vi "GetData.vi"(8 "error in (no error)":errorcluster caption="Fehler (Eingang, kein Fehler)", 10 "Name":string, 11 "Dictionary Eingang":refnum<class "Dictionary.lvclass"> caption="DNL_LabVIEW Object in") -> (0 "error out":errorcluster caption="Fehler (Ausgang)", 2 "Wert":variant, 3 "Dictionary Ausgang":refnum<class "Dictionary.lvclass"> caption="DNL_LabVIEW Object out")   [LabVIEW 2013, in "Dictionary.lvclass"]
uses:
  Dictionary.lvclass
  Dictionary.lvclass/Dictionary.ctl
  Properties/GetDict.vi
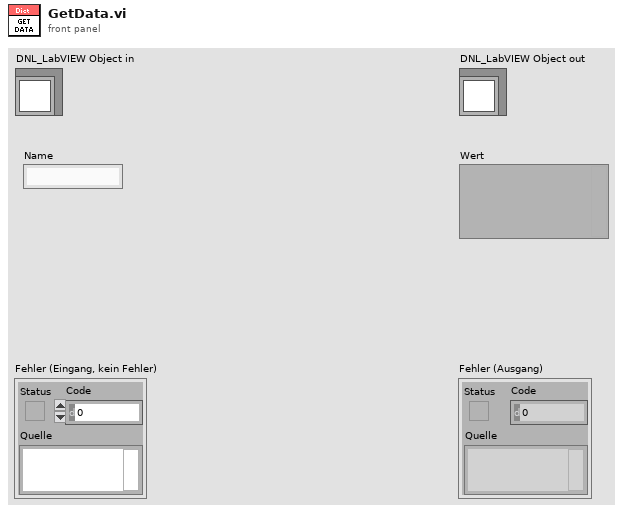
[diagram p1: front panel]
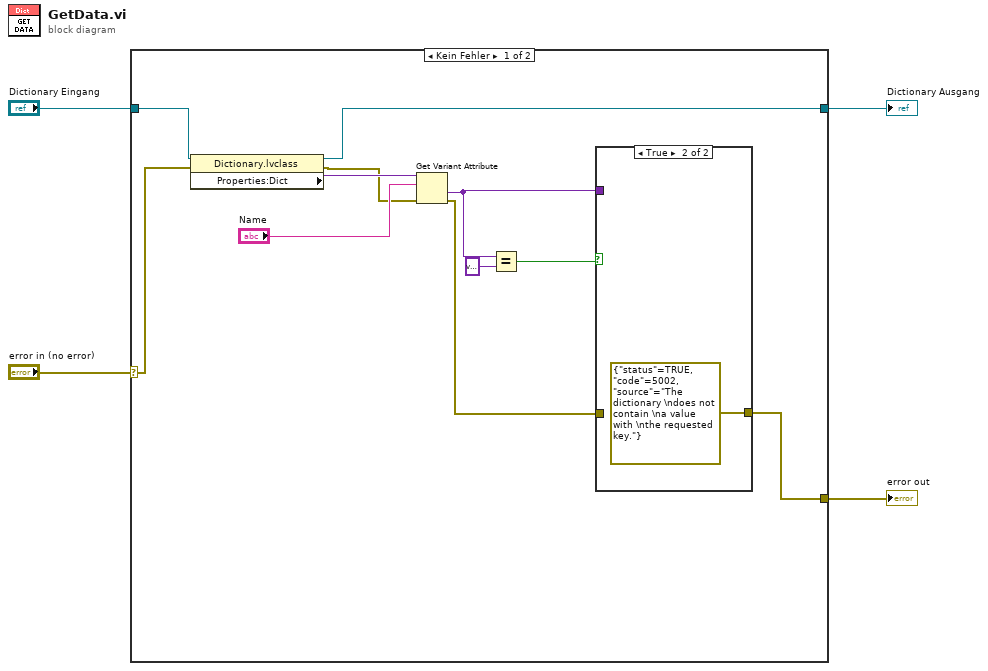
[diagram p0: block diagram]
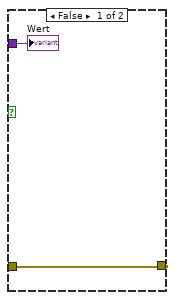
[diagram p2: hidden frame]
diagram:
  n1 = case shown="Kein Fehler" "error in (no error)" {
    selector: "error in (no error)" -> [w11 w20]
    tunnel: [w6 w20] -> w3
    tunnel: [w14 w19] -> w1
    tunnel: "Dictionary Eingang" -> [w15 w19]
    frame No Error {
      n2 = property class="Dictionary.lvclass"(reference=w15, error in=w11) -> (reference out=w14:refnum<class "Dictionary.lvclass">, error out=w10:errorcluster, "Properties:Dict"=w13:variant)
      n3 = Get Variant Attribute(Variant=w13, name="Name", error in=w10) -> (value=w5:variant, error out=w7:errorcluster)  [unwired: 1 in, 2 out]
      n4 = Equal?(x=w5, y=variant) -> (x = y?=w8:bool)
      n5 = case shown="True" w8 {
        tunnel: w7 -> [w17 _]
        tunnel: [w17 errorcluster {"status"=TRUE, "code"=5002, "source"="The dictionary \ndoes not contain \na value with \nthe requested key."} ("error out")] -> w6
        tunnel: w5 -> [w16 _]
        frame False {
          "Wert" <- w16
        }
        frame True {
        }
      }
    }
    frame Error {
    }
  }
  "error out" <- w3
  "Dictionary Ausgang" <- w1
